vi "Result.Remove Name-Value Items with Empty Values.vi"(9 "Values In":string[](array[string]), 11 "Names In":string[](array[string])) -> (1 "Values":string[](array[string]), 3 "Names":string[](array[string]))   [LabVIEW 2019]
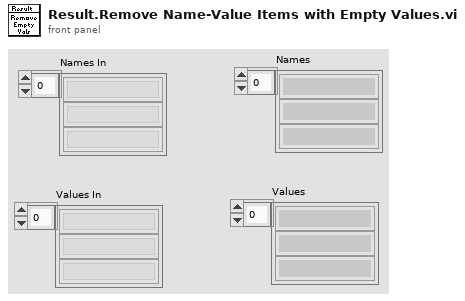
[diagram p1: front panel]
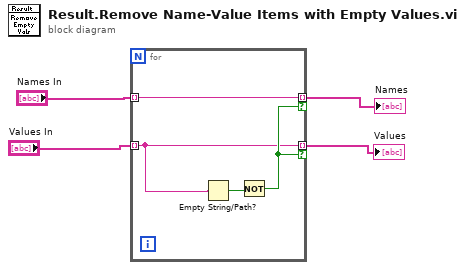
[diagram p0: block diagram]
diagram:
  n1 = for {
    tunnel: "Names In" -> [w7] mode=indexing
    tunnel: "Values In" -> [w5] mode=indexing
    tunnel: [w7] -> w2 mode=indexing if=w6
    tunnel: [w5] -> w1 mode=indexing if=w6
    n2 = Empty String/Path?(string/path=w5) -> (empty?=w8:bool)
    n3 = Not(x=w8) -> (.not. x?=w6:bool)
  }
  "Names" <- w2
  "Values" <- w1
